vi "Image I32 Array to U8 Array Autocontrast.vi"(8 "Error In":errorcluster, 9 "Min & Max % (Default: 5 -95)":dbl[](array[numeric])=[5.0, 95.0], 11 "I32 Image":i32[][](array[numeric])) -> (0 "Error Out":errorcluster, 3 "U8 5-95% Contrast Enhanced U8 Image":u8[][](array[numeric]))   [LabVIEW 2021, in "Image.lvlib"]
uses:
  Image.lvlib
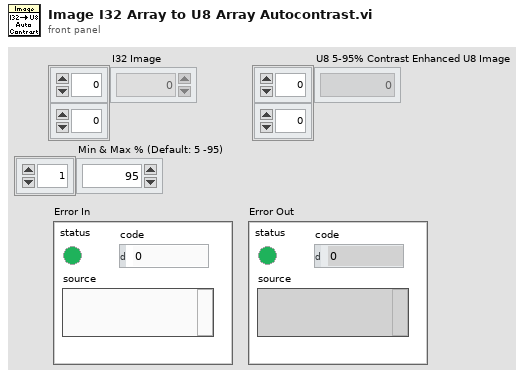
[diagram p1: front panel]
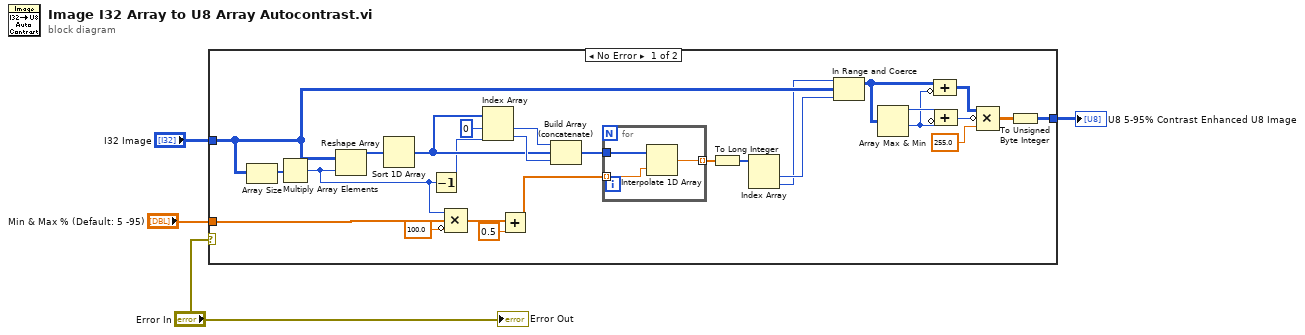
[diagram p0: block diagram]
diagram:
  n1 = case shown="No Error" "Error In" {
    tunnel: "Min & Max % (Default: 5 -95)" -> [w31 _]
    tunnel: "I32 Image" -> [w18 _]
    tunnel: [w6 _] -> w2
    frame No Error {
      n2 = Array Size(array=w18) -> (size(s)=w20:i32[])
      n3 = Multiply Array Elements(1:w20) -> (0:w19:i32)
      n4 = Reshape Array(w18, w19) -> (w21:i32[])
      n5 = Sort 1D Array(array=w21) -> (sorted array=w27:i32[])
      n6 = Decrement(x=w19) -> (x-1=w25:i32)
      n7 = Compound Arithmetic op=MULTIPLY(w19, w31, invert 100.0 ("value")) -> (w22:dbl[])
      n8 = Index Array(array=w27, index #1=0 ("index"), index #2=w25) -> (element #1=w26:i32, element #2=w28:i32)
      n9 = Add(x=w22, y=0.5) -> (x+y=w30:dbl[])
      n10 = Build Array (concatenate)(w26, w27, w28) -> (w29:i32[])
      n11 = for {
        tunnel: w29 -> [w34]
        tunnel: [w33] -> w17 mode=indexing
        tunnel: w30 -> [w32] mode=indexing
        n12 = Interpolate 1D Array(1:w32, 2:w34) -> (0:w33:dbl)
      }
      n13 = To Long Integer(number=w17) -> (32bit integer=w14:i32[])
      n14 = Index Array(array=w14) -> (element #1=w16:i32, element #2=w15:i32)  [unwired: 2 in]
      n15 = In Range and Coerce(upper limit=w15, x=w18, lower limit=w16) -> (coerced(x)=w13:i32[][])  [unwired: 1 out]
      n16 = Array Max & Min(array=w13) -> (max value=w12:i32, min value=w11:i32)  [unwired: 2 out]
      n17 = Compound Arithmetic op=ADD(w13, invert w11) -> (w8:i32[][])
      n18 = Compound Arithmetic op=ADD(w12, invert w11) -> (w10:i32)
      n19 = Compound Arithmetic op=MULTIPLY(w8, invert w10, 255.0 ("value")) -> (w7:dbl[][])
      n20 = To Unsigned Byte Integer(number=w7) -> (unsigned 8bit integer=w6:u8[][])
    }
    frame Error {
    }
  }
  "U8 5-95% Contrast Enhanced U8 Image" <- w2
  "Error Out" <- "Error In"
